vi "Preview AI Channel.vi"(7 "instance":i32, 8 "error in":errorcluster, 10 "samples":u32=2048, 11 "lia host in":refnum<class "LIA Host Interface RT.lvclass">) -> (0 "error out":errorcluster, 2 "samples":i16[](array[numeric]), 3 "lia host out":refnum<class "LIA Host Interface RT.lvclass">)   [LabVIEW 2018, in "LIA Host Interface RT.lvclass"]
uses:
  LIA Host Interface RT.lvclass
  shared/Public/message.ctl
  shared/Lock-In Amplifier Example Shared.lvlib
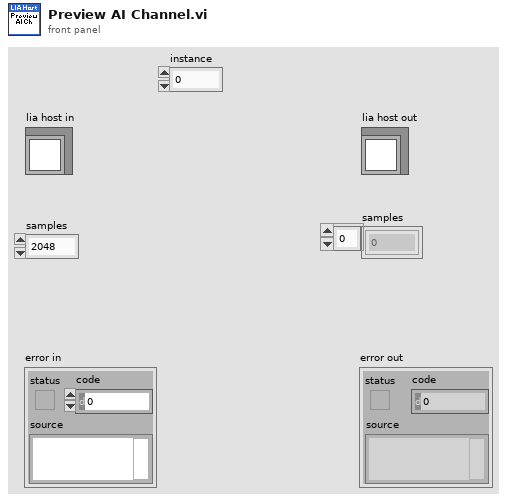
[diagram p1: front panel]
types:
  T1 = typedef "Lock-In Amplifier Example Shared.lvlib/message.ctl" = cluster{"command":u32, "payload":string}
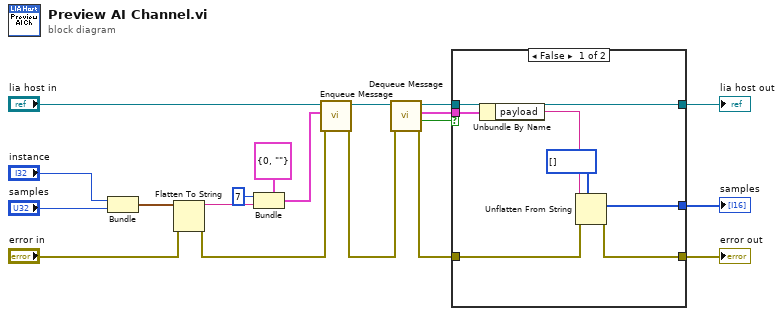
[diagram p0: block diagram]
diagram:
  n1 = Bundle("instance"="instance", "samples"="samples") -> (w14:cluster{"instance":i32, "samples":u32})  [unwired: 1 in]
  n2 = Flatten To String(anything=w14, error in (no error)="error in") -> (data string=w11:string, error out=w12:errorcluster)  [unwired: 2 in, 1 out]
  n3 = Bundle(cluster=T1 {"command"=0, "payload"=""} ("message"), "command"=u32 7, "payload"=w11) -> (w8:T1)
  n4 = call "Enqueue Message.vi"("error in"=w12, "command"=w8, "lia host in"="lia host in") -> ("error out"=w17:errorcluster, "lia host out"=w18:refnum<class "LIA Host Interface RT.lvclass">)  [unwired: 7 in]
  n5 = call "Dequeue Message.vi"("error in"=w17, "lia host in"=w18) -> ("error out"=w6:errorcluster, "timed out?"=w4:bool, "message"=w7:T1, "lia host out"=w2:refnum<class "LIA Host Interface RT.lvclass">)  [unwired: 6 in]
  n6 = case shown="False" w4 {
    tunnel: w7 -> [w26 _]
    tunnel: w6 -> [w24 w27]
    tunnel: [w22 _] -> w1
    tunnel: [w21 w27] -> w5
    tunnel: [w23 w28] -> w3
    tunnel: w2 -> [w23 w28]
    frame False {
      n7 = Unbundle By Name(w26) -> ("payload"=w25:string)
      n8 = Unflatten From String(type=i16[] [], binary string=w25, error in (no error)=w24) -> (value=w22:i16[], error out=w21:errorcluster)  [unwired: 2 in, 1 out]
    }
    frame True {
    }
  }
  "error out" <- w5
  "lia host out" <- w3
  "samples" <- w1
